vi "About.vi"() -> ()   [LabVIEW 2013]
panel:
  out "Release":string
  in  "OK":bool
  # "Rev: 1.0\nBuild Date: 09/16/2016\nReport Issue to Technical Contact: Colin.Reg@live.com"
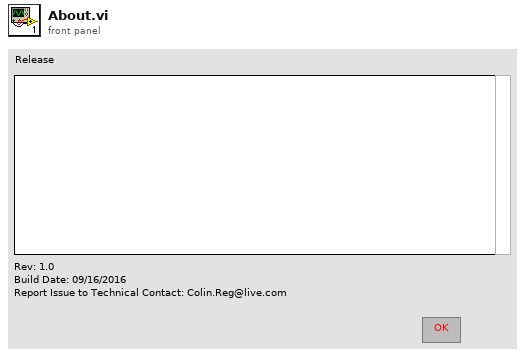
[diagram p1: front panel]
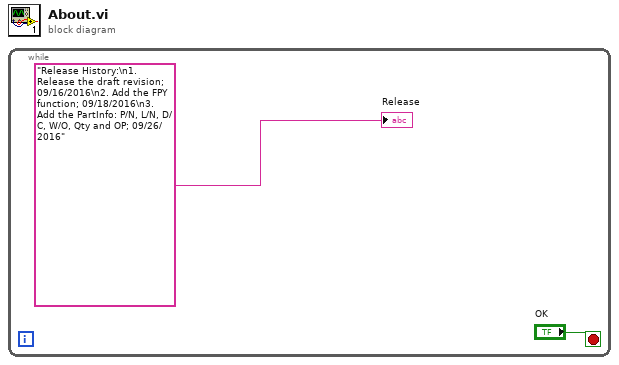
[diagram p0: block diagram]
diagram:
  n1 = while {
    stop <- "OK" stop-if-true
    "Release" <- "Release History:\n1. Release the draft revision; 09/16/2016\n2. Add the FPY function; 09/18/2016\n3. Add the PartInfo: P/N, L/N, D/C, W/O, Qty and OP; 09/26/2016"
  }
